vi "Create map data file.vi"(4 "Sample name":string, 6 "Description":string, 7 "Folder path":path, 9 "Sample holder":T2, 10 "Map parameters":T3={"B_start[T]"=0.0, "B_End[T]"=0.0, "B_rate [mT/s]"=0.0, "F_start[GHz]"=0.0, "F_end[GHz]"=0.0, "Sampling rate"=0, "Tmp [K]"=295.0, "Wait[min]"=0.0, "Points"=0, "Display signal"=enum."Phi", "Signal treat"=enum."None", "Sweep [s]"=2.0} {"Sampling rate" items=["1,1s", "2,2s", "4,5s", "9s"]}, 11 "ACQ parameters":T1 {"Enable output" items=["Disable", "Enable"]; "Amp_Mod [mV]" min=0.0 max=10000.0; "F_Mod [kHz]" min=0.1 max=100.0; "Filter order" min=1.0 max=9.0 step=1.0; "Time constant [ms]" min=0.0 max=1000.0}) -> (0 "error out":errorcluster, 3 "Byte Stream File out":refnum<file>)   [LabVIEW 2024]
uses:
  Datatypes/Map parameters.ctl
  Subsystem modules/Lock-in module/ctl/OSC sampling rate.ctl
  Datatypes/SampleHolders.ctl
  Subsystem modules/Lock-in module/ctl/MFLI parameters.ctl
  Subsystem modules/Lock-in module/Lock-in module.lvlib
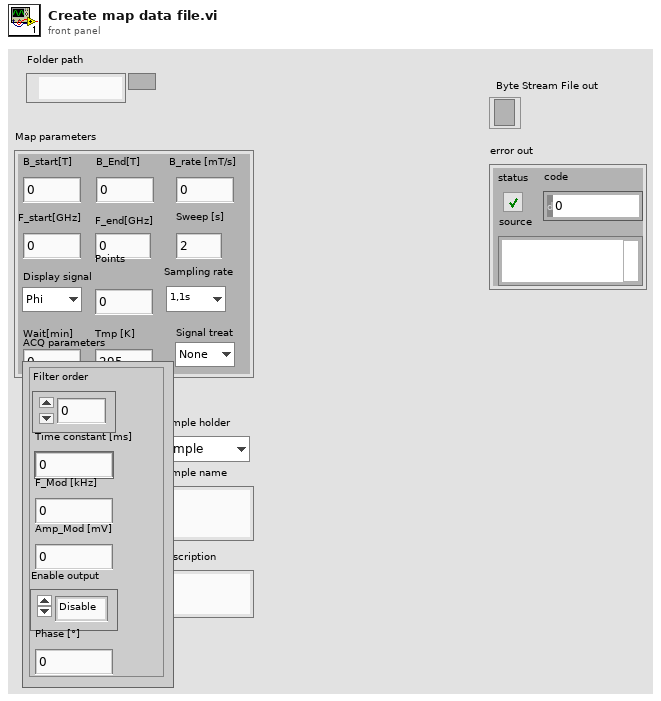
[diagram p1: front panel]
types:
  T1 = typedef "Lock-in module.lvlib/MFLI parameters.ctl" = cluster{"Filter order":dbl, "Time constant [ms]":dbl, "F_Mod [kHz]":dbl, "Amp_Mod [mV]":dbl, "Enable output":u16, "Phase [°]":dbl}
  T2 = typedef "SampleHolders.ctl" = enum16{"Simple", "Carousel", "Chip", "Rotator", "Liquid"}
  T3 = typedef "Map parameters.ctl" = cluster{"B_start[T]":dbl, "B_End[T]":dbl, "B_rate [mT/s]":dbl, "F_start[GHz]":dbl, "F_end[GHz]":dbl, "Sampling rate":T4, "Tmp [K]":dbl, "Wait[min]":dbl, "Points":u32, "Display signal":enum16{"X", "Y", "R", "Phi"}, "Signal treat":enum16{"None", "Unity norm", "Mean norm", "Standardization"}, "Sweep [s]":dbl}
  T4 = typedef "OSC sampling rate.ctl" = u16
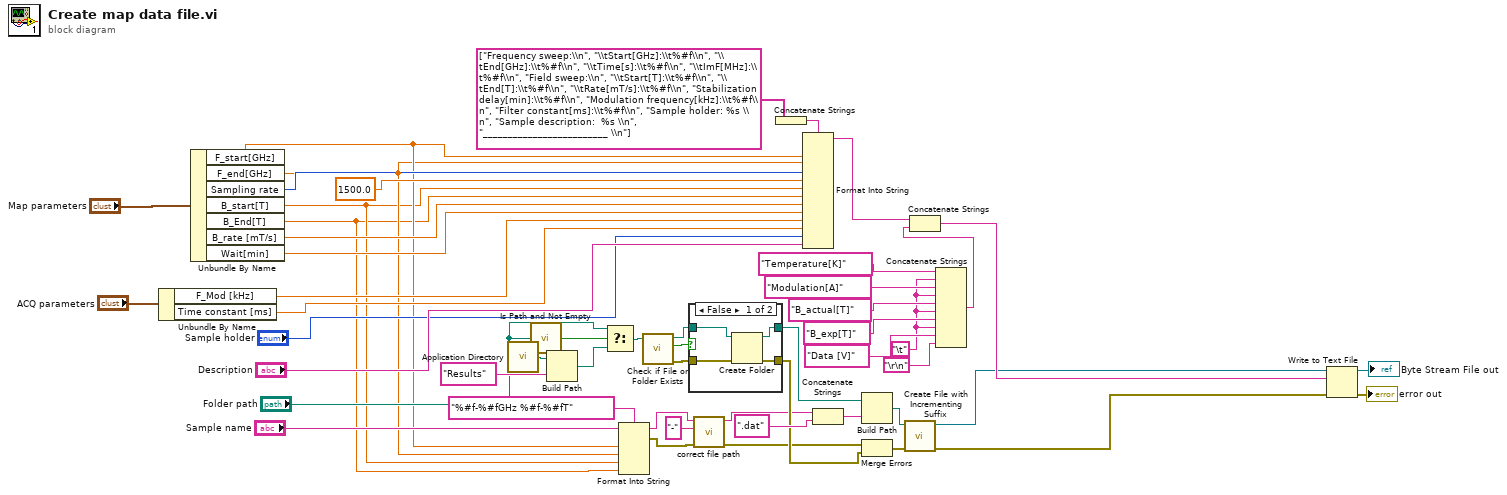
[diagram p0: block diagram]
diagram:
  w40 = "\t"
  n1 = Unbundle By Name("ACQ parameters") -> ("F_Mod [kHz]"=w51:dbl, "Time constant [ms]"=w7:dbl)
  n2 = Unbundle By Name("Map parameters") -> ("F_start[GHz]"=w6:dbl, "F_end[GHz]"=w5:dbl, "Sampling rate"=w10:T4, "B_start[T]"=w4:dbl, "B_End[T]"=w3:dbl, "B_rate [mT/s]"=w49:dbl, "Wait[min]"=w50:dbl)
  n3 = call <vilib>:"Application Directory.vi"() -> ("Application Directory"=w17:path)
  n4 = call <vilib>:"Is Path and Not Empty.vi"("path"="Folder path") -> ("Is Path and Not Empty?"=w30:bool)  [unwired: 4 in]
  n5 = Build Path(base path=w17, name or relative path="Results") -> (appended path=w32:path)
  n6 = Select(t="Folder path", s=w30, f=w32) -> (s? t:f=w31:path)
  n7 = Format Into String(format string="%#f-%#fGHz %#f-%#fT", initial string="Sample name", w6, w5, w4, w3) -> (resulting string=w21:string, error out=w26:errorcluster)  [unwired: 1 in]
  n8 = call <vilib>:"Check if File or Folder Exists.vi"("path"=w31) -> ("error out"=w28:errorcluster, "file or folder exists?"=w27:bool, "dup path"=w29:path)  [unwired: 8 in]
  n9 = case shown="False" w27 {
    tunnel: w29 -> [w54 w58]
    tunnel: [w55 w57] -> w34
    tunnel: w28 -> [w56 w57]
    tunnel: [w53 w58] -> w33
    frame False {
      n10 = Create Folder(path (use dialog)=w54, error in=w56) -> (created path=w53:path, error out=w55:errorcluster)  [unwired: 1 in, 1 out]
    }
    frame True {
    }
  }
  n11 = call "correct file path.vi"("error in (no error)"=w26, "replacement (-)"="-" ("replacement"), "input path"=w21) -> ("error out"=w24:errorcluster, "corrected path"=w20:string)  [unwired: 7 in]
  n12 = Concatenate Strings(string[] ["Frequency sweep:\\n", "\\tStart[GHz]:\\t%#f\\n", "\\tEnd[GHz]:\\t%#f\\n", "\\tTime[s]:\\t%#f\\n", "\\tImF[MHz]:\\t%#f\\n", "Field sweep:\\n", "\\tStart[T]:\\t%#f\\n", "\\tEnd[T]:\\t%#f\\n", "\\tRate[mT/s]:\\t%#f\\n", "Stabilization delay[min]:\\t%#f\\n", "Modulation frequency[kHz]:\\t%#f\\n", "Filter constant[ms]:\\t%#f\\n", "Sample holder: %s \\n", "Sample description:  %s \\n", "_________________________ \\n"]) -> (w15:string)
  n13 = Format Into String(format string=w15, w6, w5, w10, 1500.0 ("input 4"), w4, w3, w49, w50, w51, w7, "Sample holder", "Description") -> (resulting string=w14:string)  [unwired: 2 in, 1 out]
  n14 = Concatenate Strings(w20, ".dat" ("string")) -> (w22:string)
  n15 = Build Path(base path=w33, name or relative path=w22) -> (appended path=w23:path)
  n16 = Merge Errors(w24, w34) -> (w25:errorcluster)
  n17 = call <vilib>:"Create File with Incrementing Suffix.vi"("error in (no error)"=w25, "file path"=w23) -> ("error out"=w1:errorcluster, "refnum out"=w2:refnum<file>)  [unwired: 7 in, 1 out]
  n18 = Concatenate Strings("Temperature[K]", w40, "Modulation[A]", w40, "B_actual[T]" ("string"), w40, "B_exp[T]", w40, "Data [V]", "\r\n") -> (w18:string)
  n19 = Concatenate Strings(w14, w18) -> (w19:string)
  n20 = Write to Text File(file (use dialog)=w2, text=w19, error in=w1) -> (refnum out=→"Byte Stream File out":refnum<file>, error out=→"error out":errorcluster)  [unwired: 1 in, 1 out]
